vi "SP Read Single.vi"(8 "error in":errorcluster, 9 "Channel Index":i32=1, 11 "Flow Setpoint in":refnum<class "Flow Setpoint.lvclass">) -> (0 "error out":errorcluster, 1 "Changed or First Call?":bool, 2 "Flow SP":dbl, 3 "Flow Setpoint out":refnum<class "Flow Setpoint.lvclass">)   [LabVIEW 2023, in "Flow Setpoint.lvclass"]
uses:
  Flow Setpoint.lvclass
  Flow Setpoint.lvclass/Flow Setpoint.ctl
  Parents/Setpoint/Setpoint.lvclass
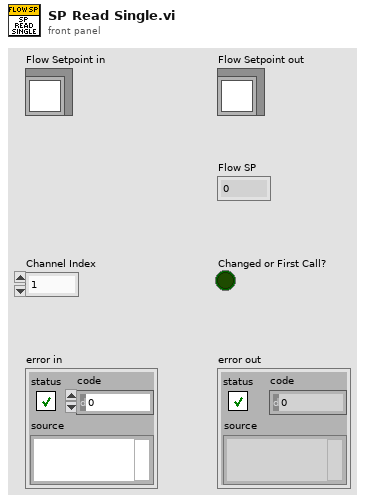
[diagram p1: front panel]
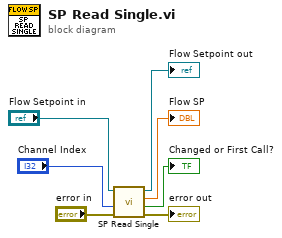
[diagram p0: block diagram]
diagram:
  n1 = call-parent "SP Read Single.vi"("error in"="error in", "Channel Index"="Channel Index", "Setpoint in"="Flow Setpoint in") -> ("error out"=→"error out":errorcluster, "Changed or First Call?"=→"Changed or First Call?":bool, "Current SP"=→"Flow SP":dbl, "Setpoint out"=→"Flow Setpoint out":refnum<class "Flow Setpoint.lvclass">)  [unwired: 5 in]
